vi "RSZVB Set Reference Receiver After First Cal Sweep.vi"(7 "Fast Source Power Calibration (F: Off)":bool, 8 "error in (no error)":errorcluster {"code" format="%.0x"}, 9 "Port Number (1)":i32=1, 10 "Channel (1)":i32=1, 11 "VISA session":refnum<visa-resource-name>) -> (0 "error out":errorcluster {"code" format="%.0x"}, 3 "dup VISA session":refnum<visa-resource-name>)   [LabVIEW 2011]
doc: "This VI enables or disables a fast source power calibration, where the external power meter is used for the first calibration sweep only. \n\nRemote-control command(s):\nSOURce<Ch>:POWer<Pt>:CORRection:FAST ON | OFF"
uses:
  _utility/RSZVB Global Data.vi
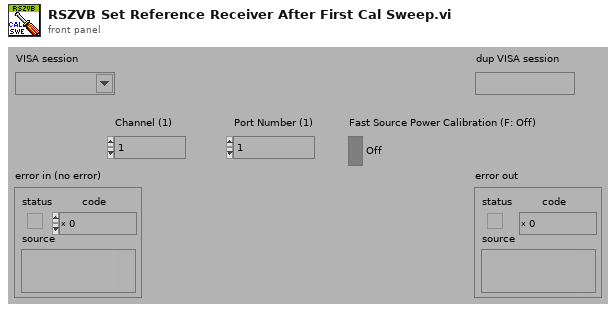
[diagram p1: front panel]
types:
  T1 = cluster{"Error Checking (T: On)":bool, "Installed Options":string[], "Data Valid?":bool, "Ports":i32, "Model":string[], "Option Checking (T: On)":bool}[]
  T2 = cluster{"Error Checking (T: On)":bool, "Installed Options":string[], "Data Valid?":bool, "Ports":i32, "Model":string[], "Option Checking (T: On)":bool}
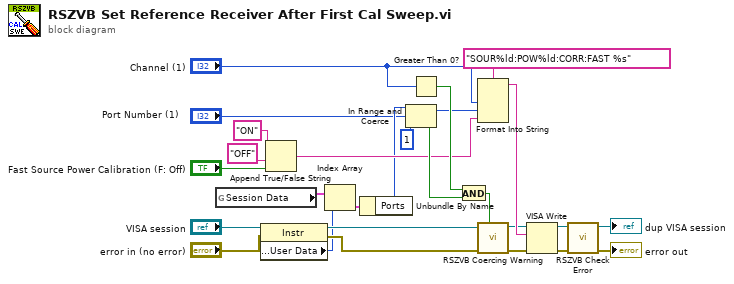
[diagram p0: block diagram]
diagram:
  n1 = global read "RSZVB Global Data.vi" "Session Data"() -> (w14:T1)
  n2 = property class="Instr"(reference="VISA session", error in="error in (no error)") -> (reference out=w16:refnum<visa-resource-name>, error out=w27:errorcluster, "General Settings:User Data"=w13:u32)
  n3 = Append True/False String(1:"Fast Source Power Calibration (F: Off)", 2:"OFF" ("false string"), 3:"ON" ("true string")) -> (0:w20:string)  [unwired: 1 in]
  n4 = Index Array(array=w14, index=w13) -> (element=w15:T2)
  n5 = Unbundle By Name(w15) -> ("Ports"=w17:i32)
  n6 = In Range and Coerce(upper limit=w17, x="Port Number (1)", lower limit=1) -> (coerced(x)=w19:i32, In Range?=w24:bool)
  n7 = Greater Than 0?(x="Channel (1)") -> (x > 0?=w25:bool)
  n8 = And(x=w25, y=w24) -> (x .and. y?=w21:bool)
  n9 = Format Into String(format string="SOUR%ld:POW%ld:CORR:FAST %s", "Channel (1)", w19, w20) -> (resulting string=w26:string)  [unwired: 2 in, 1 out]
  n10 = call "RSZVB Coercing Warning.vi"("In Range?"=w21, "error in (no error)"=w27, "VISA session"=w16) -> ("error out"=w10:errorcluster, "dup VISA session"=w22:refnum<visa-resource-name>)  [unwired: 7 in]
  n11 = VISA Write(VISA resource name=w22, write buffer=w26, error in (no error)=w10) -> (VISA resource name out=w23:refnum<visa-resource-name>, error out=w11:errorcluster)  [unwired: 1 out]
  n12 = call "RSZVB Check Error.vi"("error in (no error)"=w11, "VISA session"=w23) -> ("error out"=→"error out":errorcluster, "dup VISA session"=→"dup VISA session":refnum<visa-resource-name>)  [unwired: 8 in]
